vi "Comic_Crawler_Main_UI.vi"(11 "manager_daemon":refnum<class "manager_daemon.lvclass">) -> ()   [LabVIEW 2024]
uses:
  comic_crawler_class/status--cluster.ctl
  CV_downloader/status--cluster.ctl
  comic_manager/manager_daemon/manager_daemon.lvclass
  comic_crawler_class/comic_crawler.lvclass
  CV_downloader/CV_downloader.lvclass
  <vilib>/addons/_JKI Toolkits/State Machine/_JKI_lib_State_Machine.llb/Select State(s)_err__jki_lib_state_machine.vi
  003bbeb0-736b-424c-b7a2-e9a572b8fb0f.vi
  <vilib>/addons/_JKI Toolkits/State Machine/_JKI_lib_State_Machine.llb/Periodic Trigger__ogtk__JKI-SM__jki_lib_state_machine.vi
panel:
  out "added URLs":string[](array[string])
  in  "Add URL":bool
  in  "volume url":string
  out "manager status":T1
  out "size(s)":i32
  out "out of date filelist":path[](array[path])
  in  "Stop Crawler":bool
  in  "Start Crawler":bool
  out "crawler status":T2
  in  "search dirs":path[](array[path])=[path "D:/Comics/data/cv_volumes"]
  in  "Exit":bool
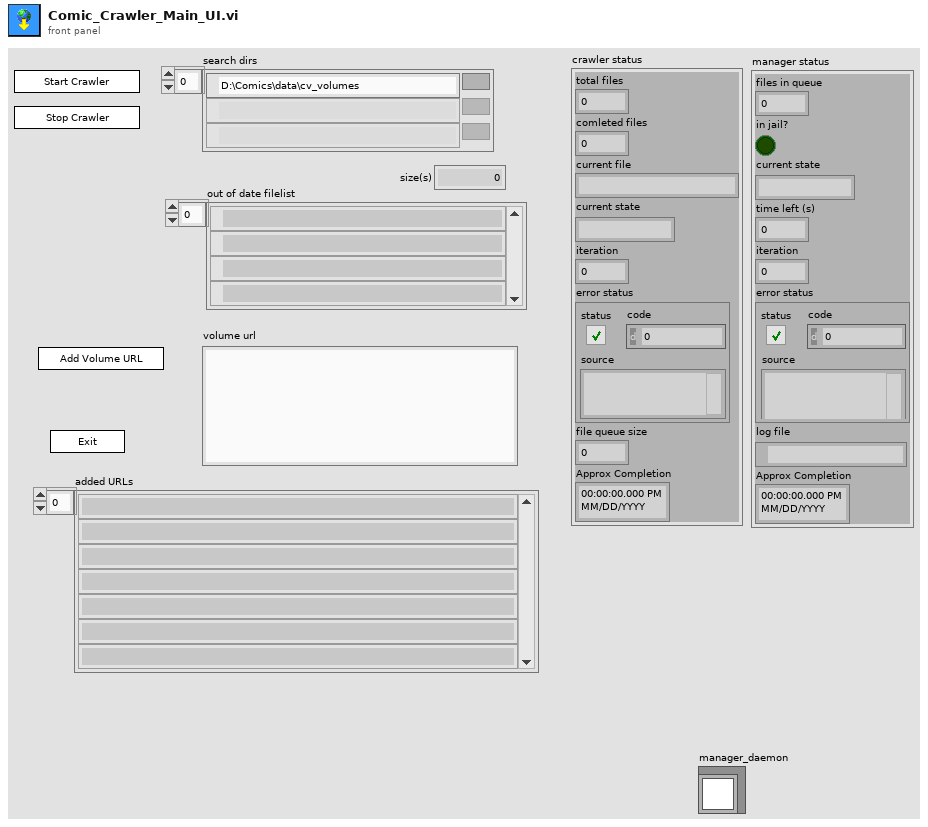
[diagram p1: front panel]
types:
  T1 = typedef "CV_downloader.lvclass/status--cluster.ctl" = cluster{"files in queue":i32, "in jail?":bool, "current state":string, "time left (s)":dbl, "iteration":i32, "error status":errorcluster, "log file":path, "Approx Completion":timestamp}
  T2 = typedef "comic_crawler.lvclass/status--cluster.ctl" = cluster{"total files":i32, "comleted files":i32, "current file":string, "current state":string, "iteration":i32, "error status":errorcluster, "file queue size":i32, "Approx Completion":timestamp}
  T3 = enum32{"Invalid", "Standard", "Closed", "Hidden", "Minimized", "Maximized"}
  T4 = enum32{"invalid app kind", "Development System", "Run Time System", "Student Edition", "Embedded LabVIEW", "Evaluation", "Custom"}
  T5 = cluster{"Core":cluster{"Current VI Reference":refnum<vi>, "Close Panel on Exit?":bool}, "TO":i32, "crawler":refnum<class "comic_crawler.lvclass">, "files for update":path[], "manager":refnum<class "CV_downloader.lvclass">, "vol_dir":path, "iss_dir":path, "manager_daemon":refnum<class "manager_daemon.lvclass">}
  T6 = cluster{"Current VI Reference":refnum<vi>, "Close Panel on Exit?":bool}
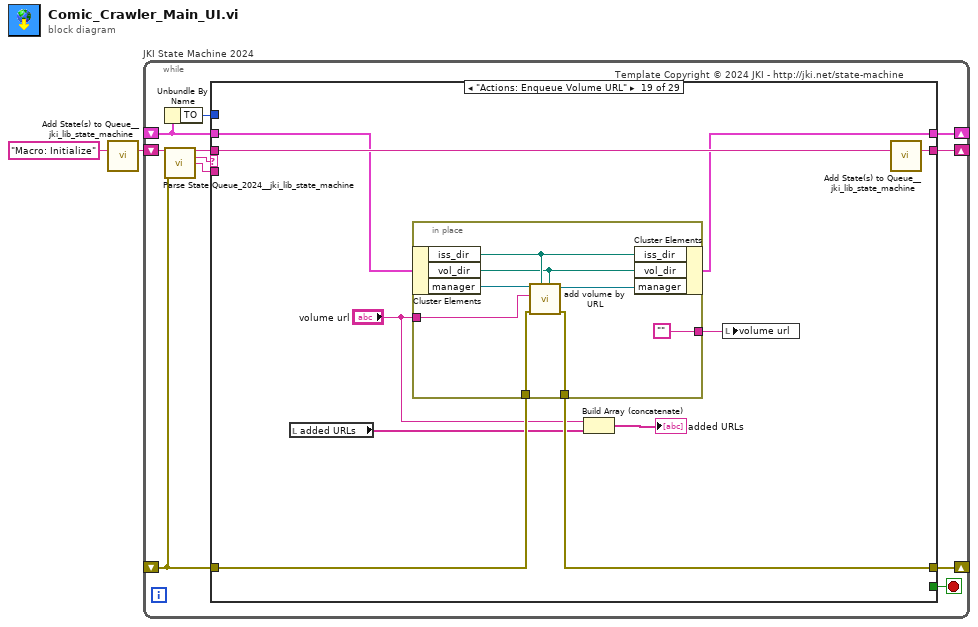
[diagram p0: block diagram]
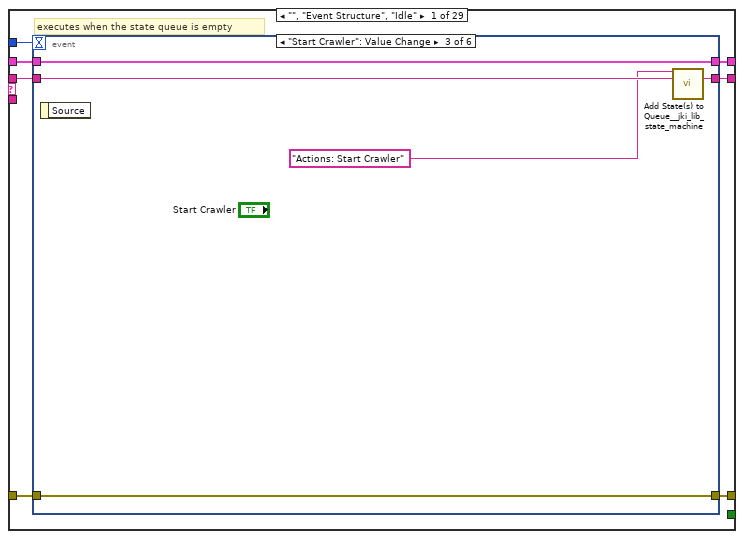
[diagram p2: hidden frame]
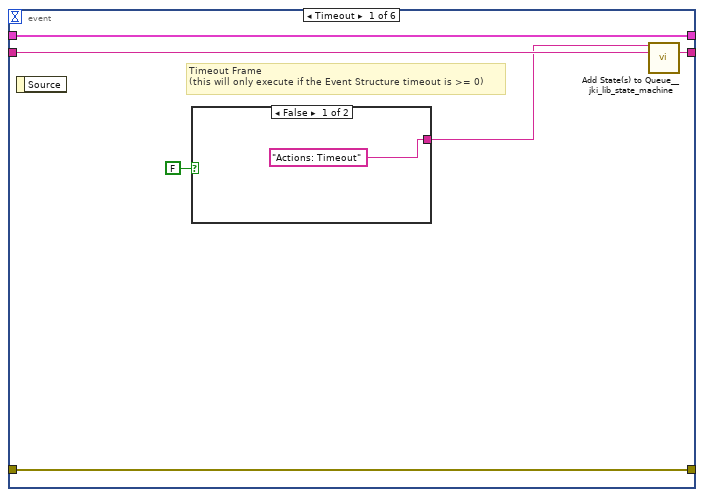
[diagram p3: hidden frame]
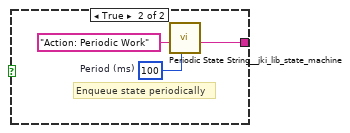
[diagram p4: hidden frame]
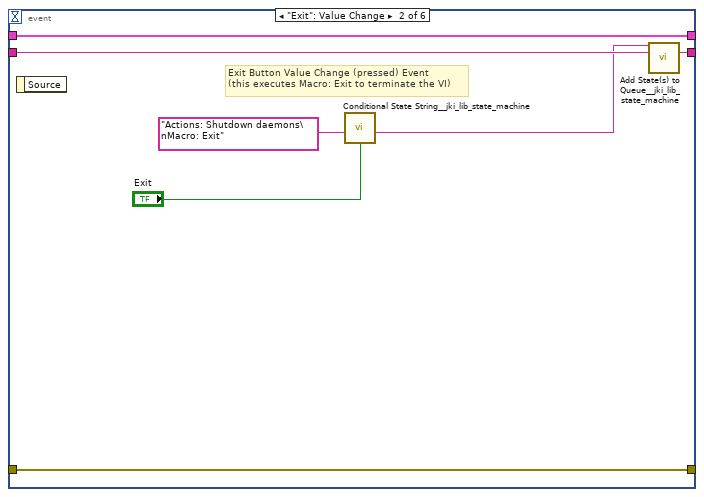
[diagram p5: hidden frame]
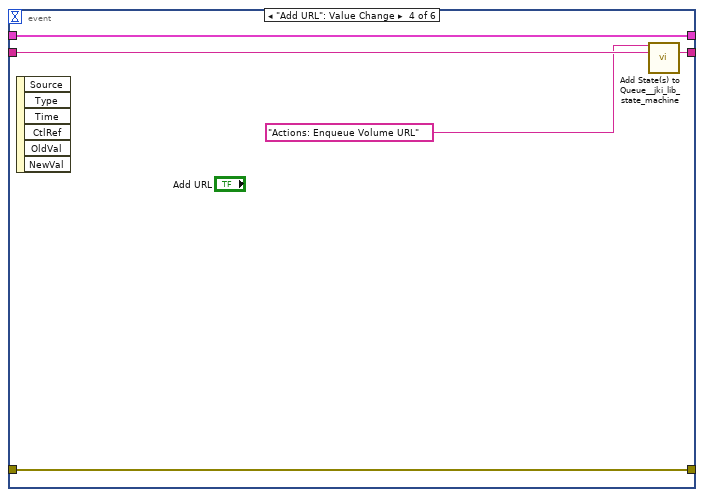
[diagram p6: hidden frame]
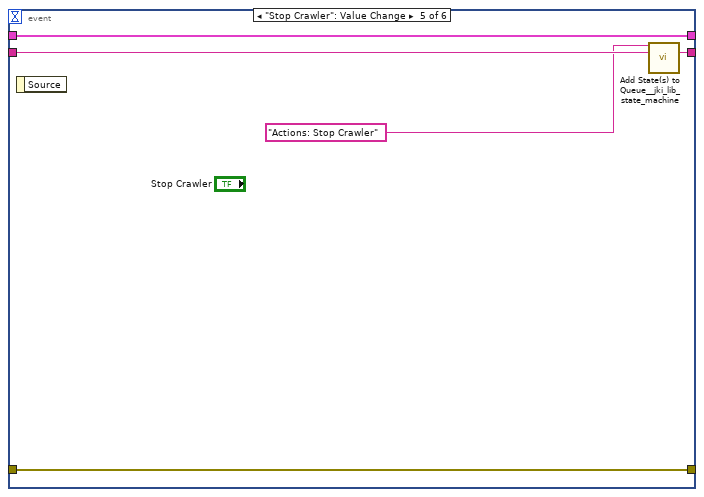
[diagram p7: hidden frame]
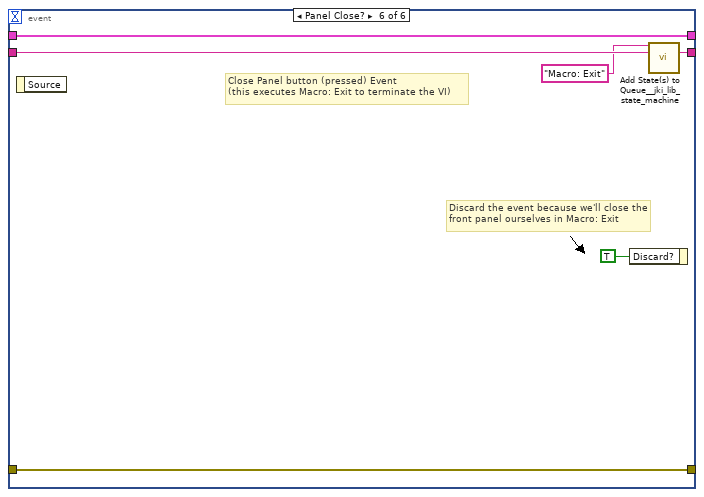
[diagram p8: hidden frame]
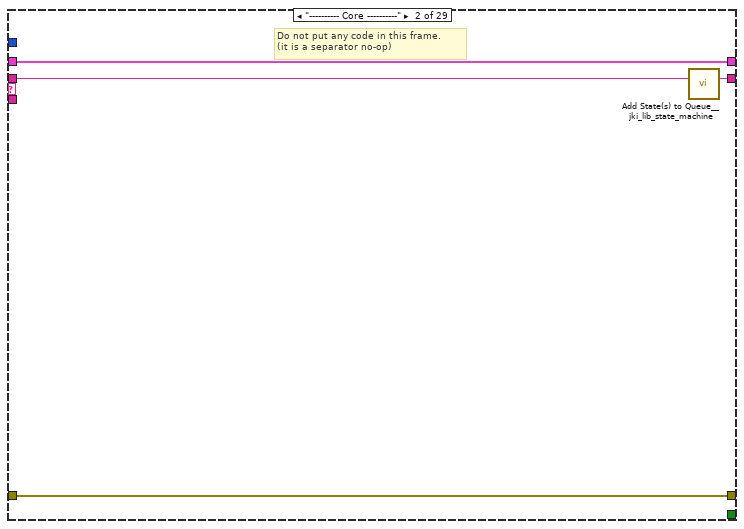
[diagram p9: hidden frame]
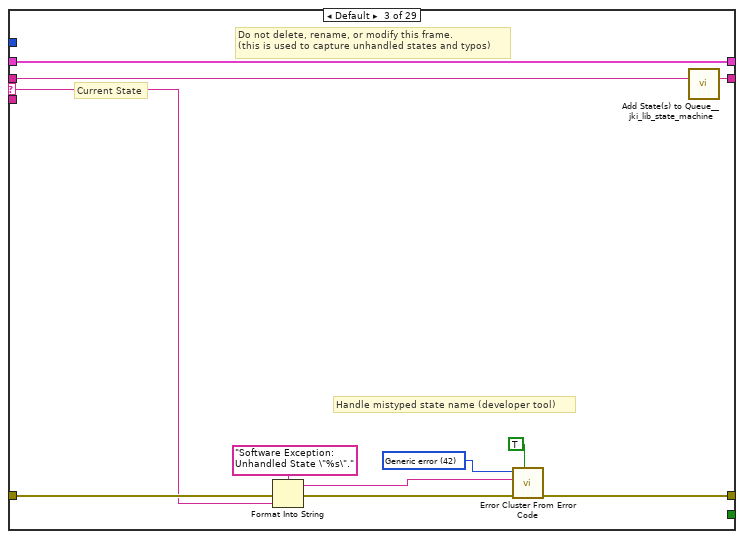
[diagram p10: hidden frame]
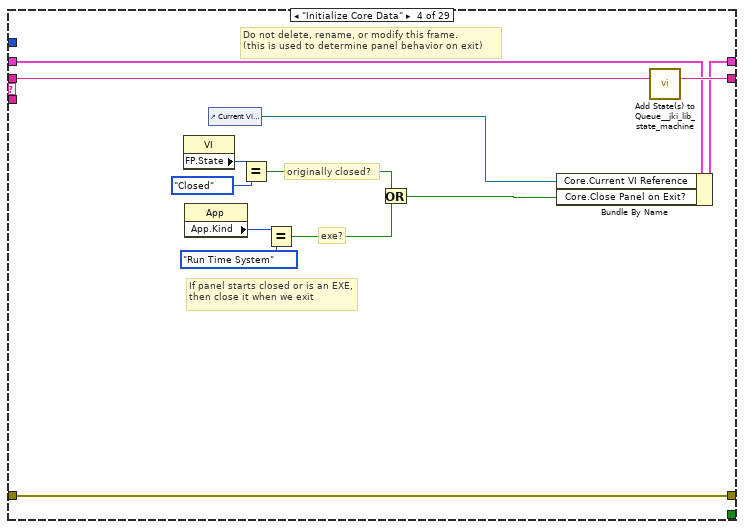
[diagram p11: hidden frame]
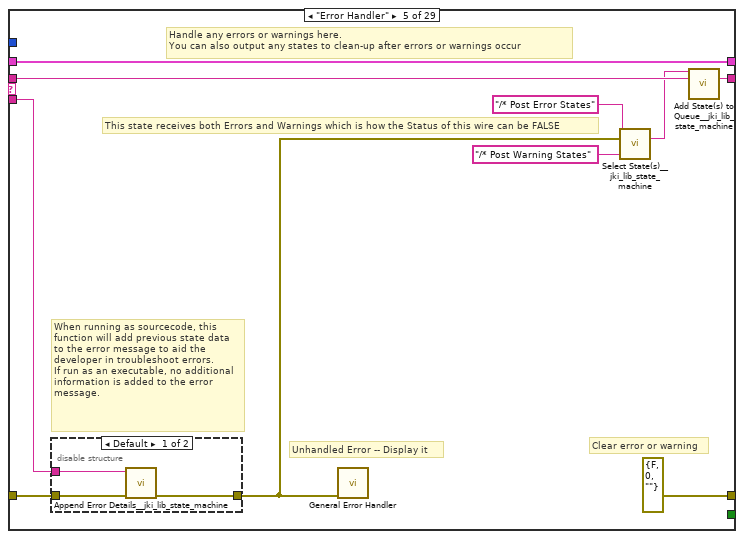
[diagram p12: hidden frame]
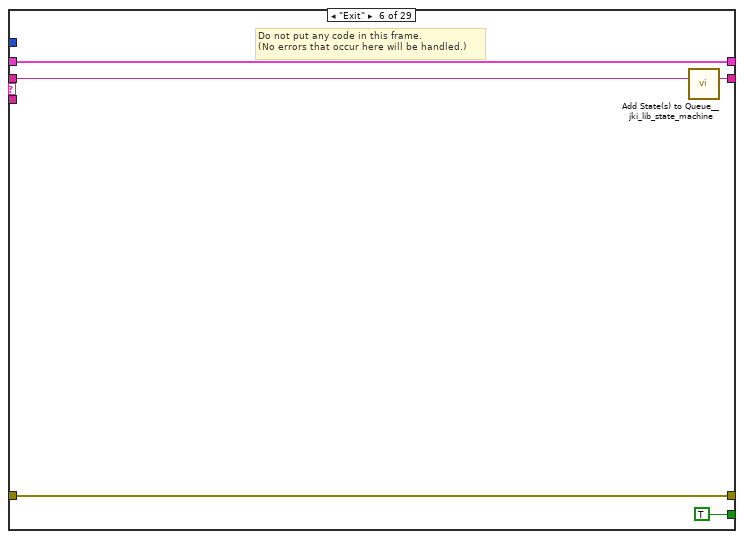
[diagram p14: hidden frame]
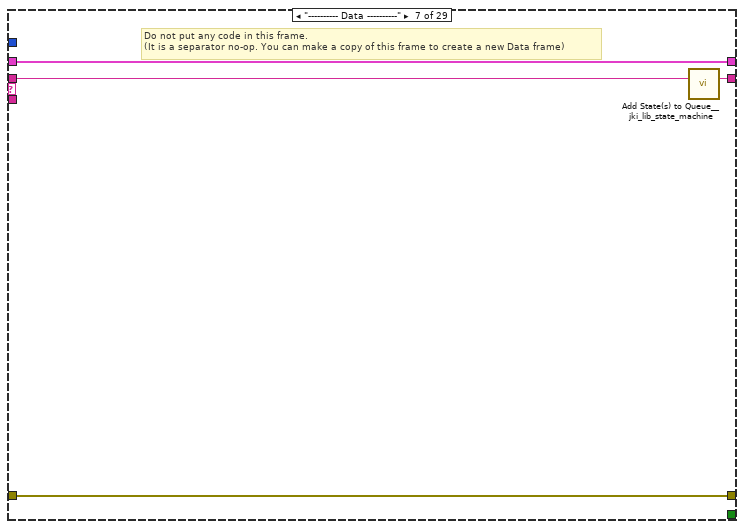
[diagram p15: hidden frame]
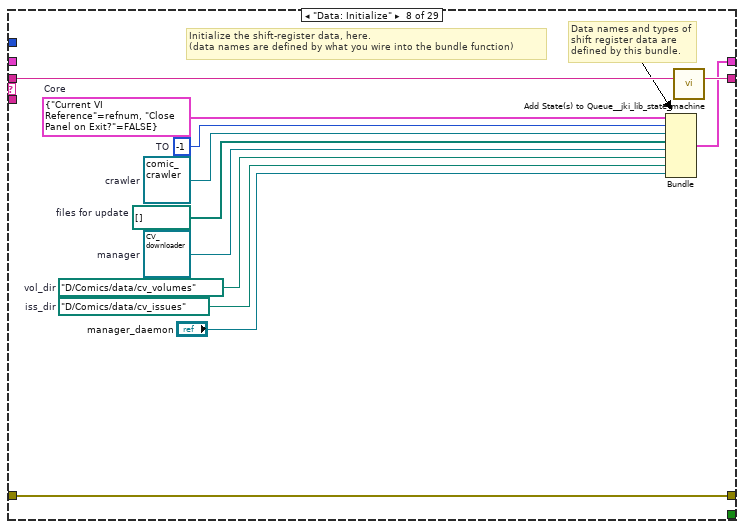
[diagram p16: hidden frame]
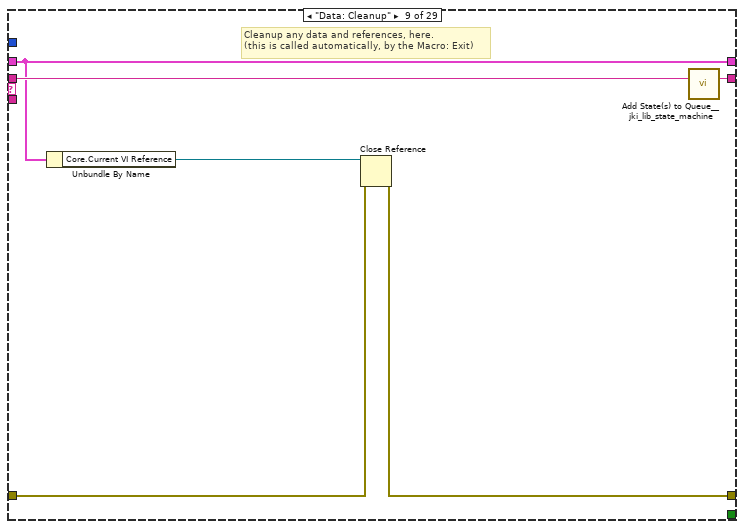
[diagram p17: hidden frame]
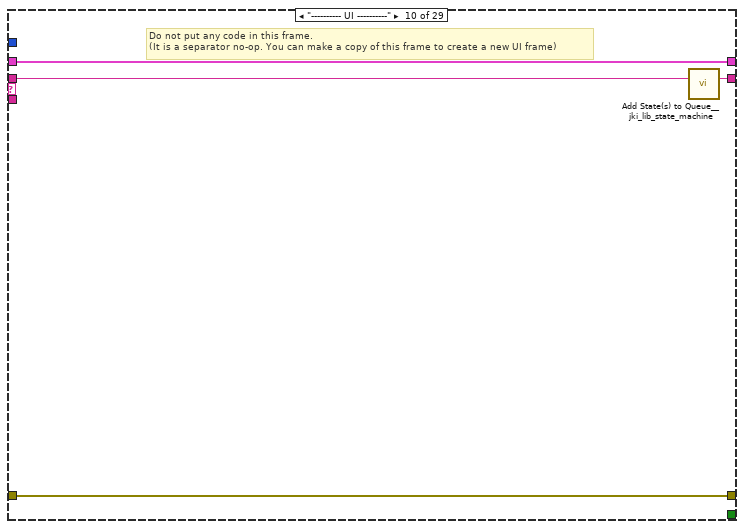
[diagram p18: hidden frame]
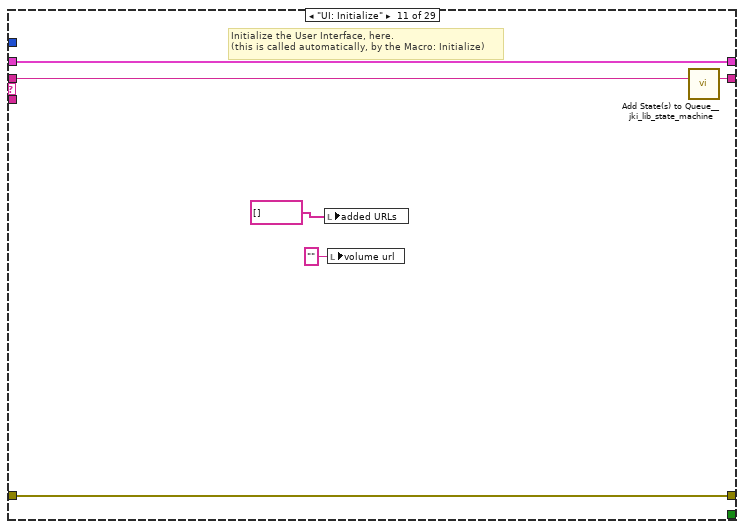
[diagram p19: hidden frame]
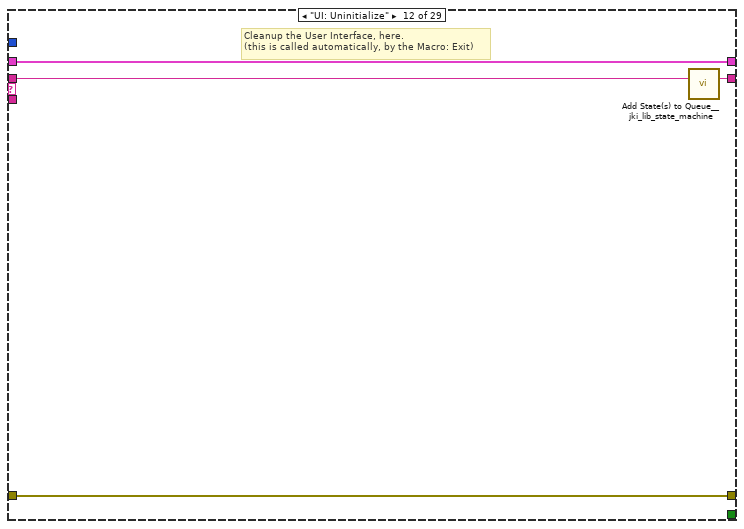
[diagram p20: hidden frame]
diagram:
  n1 = call <vilib>:"Add State(s) to Queue__jki_lib_state_machine.vi"("State(s) in (\"\")"="Macro: Initialize") -> ("States Out"=w2:string)  [unwired: 14 in]
  n2 = while "JKI State Machine 2024" {
    shift-right: [w6] -> _
    shift-left: _ -> [w4]
    shift-right: [w9] -> _
    shift-left: _ -> [w5]
    shift-right: [w8] -> _
    shift-left: w2 -> [w10]
    stop <- w7 stop-if-true
    # "Template Copyright © 2024 JKI - http://jki.net/state-machine"
    n3 = Unbundle By Name(w4) -> ("TO"=w3:i32)
    n4 = call <vilib>:"Parse State Queue_2024__jki_lib_state_machine.vi"("State Queue"=w10, "Error In (no error)"=w5) -> ("Remaining States"=w12:string, "Current State"=w13:string, "Arguments"=w11:string)  [unwired: 11 in]
    n5 = case shown="\"Actions: Enqueue Volume URL\"" w13 {
      selector: w13 -> [_ _ w63 _ _ _ _ _ _ _ _ _ _ _ _ _ _ _ _ _ _ _ _ _ _ _ _ _ _]
      tunnel: w12 -> [w20 w62 w67 w86 w96 w105 w109 w121 w127 w131 w137 w141 w147 w158 w227 w232 w241 w245 w255 w267 w276 w286 w293 w305 w318 w332 w348 w361 w373]
      tunnel: w11 -> [_ _ _ _ w91 _ _ _ _ _ _ _ w142 w152 _ _ _ _ _ _ _ _ _ _ _ _ _ _ _]
      tunnel: w4 -> [w18 w59 w65 w79 w93 w103 w106 _ w122 w128 w135 w139 w145 w154 w224 w229 w239 w242 w253 w264 w273 w280 w291 w303 w316 w330 w346 w358 w371]
      tunnel: [w17 w60 w69 w83 errorcluster {"status"=FALSE, "code"=0, "source"=""} ("error out") w102 w107 w118 w123 w129 w134 w138 w143 w155 w225 w230 w236 w243 w252 w265 w270 w282 w288 w300 w313 w325 w343 w354 w368] -> w9
      tunnel: w5 -> [w14 w60 w68 w83 w92 w102 w107 w118 w124 w129 w134 w138 w144 w156 w225 w230 w236 w243 w251 w265 w274 w283 w289 w301 w314 w328 w344 w357 w369]
      tunnel: [w19 w61 w66 w85 w95 w104 w108 w120 w126 w130 w136 w140 w146 w157 w226 w231 w240 w244 w254 w266 w275 w285 w292 w304 w317 w331 w347 w360 w372] -> w8
      tunnel: [_ _ _ _ _ TRUE _ _ _ _ _ _ _ _ _ _ _ _ _ _ _ _ _ _ _ _ _ _ _] -> w7
      tunnel: [w16 w59 w65 w84 w93 w103 w106 w119 w122 w128 w135 w139 w145 w154 w224 w229 w239 w242 w250 w264 w272 w284 w290 w302 w315 w329 w345 w358 w370] -> w6
      tunnel: w3 -> [w15 _ _ _ _ _ _ _ _ _ _ _ _ _ _ _ _ _ _ _ _ _ _ _ _ _ _ _ _]
      frame "", "Event Structure", "Idle" {
        # "executes when the state queue is empty"
        n6 = event shown="[2] \"Start Crawler\": Value Change" {
          selector: _ -> [_ _ _ _ _ _]
          dyn-events: _ -> [_ _ _ _ _ _]
          timeout: w15 -> [_ _ _ _ _ _]
          tunnel: w20 -> [w26 w37 w42 w47 w52 w58]
          tunnel: [w25 w36 w41 w46 w51 w57] -> w19
          tunnel: w18 -> [w23 w34 w39 w44 w49 w55]
          tunnel: [w24 w35 w40 w45 w50 w56] -> w17
          tunnel: w14 -> [w24 w35 w40 w45 w50 w56]
          tunnel: [w23 w34 w39 w44 w49 w55] -> w16
          event Timeout {
            # "Timeout Frame\n(this will only execute if the Event Structure timeout is >= 0)"
            n7 = event-data() -> ()  [unwired: 1 in, 1 out]
            n8 = case shown="False" FALSE {
              tunnel: ["Actions: Timeout" ("State Out") w30] -> w22
              frame False {
              }
              frame True {
                w28 = u32 100  # Period (ms)
                # "Enqueue state periodically"
                n9 = call <vilib>:"Periodic State String__jki_lib_state_machine.vi"("Period (ms)"=w28, "State"="Action: Periodic Work") -> ("State Out"=w30:string)  [unwired: 9 in]
              }
            }
            n10 = call <vilib>:"Add State(s) to Queue__jki_lib_state_machine.vi"("State(s) in Front (\"\")"=w22, "State(s) in (\"\")"=w26) -> ("States Out"=w25:string)  [unwired: 13 in]
          }
          event "Exit": Value Change {
            # "Exit Button Value Change (pressed) Event\n(this executes Macro: Exit to terminate the VI)"
            n11 = event-data() -> ()  [unwired: 1 in, 1 out]
            n12 = call <vilib>:"Conditional State String__jki_lib_state_machine.vi"("Do State(s)?"="Exit", "State"="Actions: Shutdown daemons\nMacro: Exit") -> ("State Out"=w31:string)  [unwired: 7 in]
            n13 = call <vilib>:"Add State(s) to Queue__jki_lib_state_machine.vi"("State(s) in Front (\"\")"=w31, "State(s) in (\"\")"=w37) -> ("States Out"=w36:string)  [unwired: 13 in]
          }
          event "Start Crawler": Value Change {
            n14 = event-data() -> ()  [unwired: 1 in, 1 out]
            n15 = call <vilib>:"Add State(s) to Queue__jki_lib_state_machine.vi"("State(s) in Front (\"\")"="Actions: Start Crawler", "State(s) in (\"\")"=w42) -> ("States Out"=w41:string)  [unwired: 13 in]
          }
          event "Add URL": Value Change {
            n16 = event-data() -> ()  [unwired: 1 in, 6 out]
            n17 = call <vilib>:"Add State(s) to Queue__jki_lib_state_machine.vi"("State(s) in Front (\"\")"="Actions: Enqueue Volume URL", "State(s) in (\"\")"=w47) -> ("States Out"=w46:string)  [unwired: 13 in]
          }
          event "Stop Crawler": Value Change {
            n18 = event-data() -> ()  [unwired: 1 in, 1 out]
            n19 = call <vilib>:"Add State(s) to Queue__jki_lib_state_machine.vi"("State(s) in Front (\"\")"="Actions: Stop Crawler", "State(s) in (\"\")"=w52) -> ("States Out"=w51:string)  [unwired: 13 in]
          }
          event Panel Close? {
            # "Discard the event because we'll close the front panel ourselves in Macro: Exit"
            # "Close Panel button (pressed) Event\n(this executes Macro: Exit to terminate the VI)"
            n20 = event-data() -> ()  [unwired: 1 in, 1 out]
            n21 = event-data("Discard?"=TRUE) -> ()  [unwired: 1 in, 1 out]
            n22 = call <vilib>:"Add State(s) to Queue__jki_lib_state_machine.vi"("State(s) in Front (\"\")"="Macro: Exit", "State(s) in (\"\")"=w58) -> ("States Out"=w57:string)  [unwired: 13 in]
          }
        }
      }
      frame "---------- Core ----------" {
        # "Do not put any code in this frame.\n(it is a separator no-op)"
        n23 = call <vilib>:"Add State(s) to Queue__jki_lib_state_machine.vi"("State(s) in (\"\")"=w62) -> ("States Out"=w61:string)  [unwired: 14 in]
      }
      frame Default {
        w72 = 42 items=["No error", "Argument error", "Memory is full", "Out of zone", "End of file", "File already open", "Generic file I/O error", "File not found", "File permission error", "Disk is full", "Duplicate path", "Too many files open", "System feature not enabled", "Resource file not found", "Cannot add resource", "Resource not found", "Image not found", "Image memory error", "Pen does not exist", "Config type invalid", "Config token not found", "Config parse error", "Config memory error", "Bad external code format", "Bad external code offset", "External code not present", "Null window", "Destroy window error", "Null menu", "Print aborted", "Bad print record", "Print driver error", "Windows error during printing", "Memory error during printing", "Print dialog error", "Generic print error", "Invalid device refnum", "Device not found", "Device parameter error", "Device unit error", "Cannot open device", "Device call aborted", "Generic error", "Cancelled by user", "Object ID too low", "Object ID too high", "Object not in heap", "Unknown heap", "Unknown object (invalid DefProc)", "Unknown object (DefProc not in table)", "Message out of range", "Invalid (null) method", "Unknown message", "Manager call not supported", "Bad address", "Network operation in progress", "Network operation timed out", "Connection is busy", "Network attribute not supported", "Network error", "Address in use", "System out of memory", "Connection aborted", "Connection refused", "Not connected", "Already connected", "Connection closed", "Initialization error (interapplication manager)", "Bad occurrence", "Wait on unbound occurrence handler", "Occurrence queue overflow", "Datalog type conflict", "Unused", "Unrecognized type (interapplication manager)", "Memory corrupt", "Failed to make temporary DLL", "Old CIN version", "Drag socket not found", "Failed to load drop-object", "Failed to register OLE object", "Failed to release OLE object", "Format specifier type mismatch", "Unknown format specifier", "Too few format specifiers", "Too many format specifiers", "Scan failed", "Newer CIN version", "Error converting to variant", "Runtime menu error", "Password tampered", "Variant attribute not found", "Incompatible variant data type", "Event data is not available", "Event Store is not present", "Occurrence is not found", "Event Queue is not created", "Event info is not available", "Refnum passed is NULL", "Error retrieving Class GUID", "Error retrieving CoClass GUID", "Error retrieving TypeLib GUID.", "Bad built application magic bytes.", "Specific driver is different from the specific driver associated with the Logical Name.", "There is no session opened to the class driver.", "Max Error", "MAX - Error with config objects", "MAX - Error loading configuration", "MAX - Group not supported"]
        # "Current State"
        # "Do not delete, rename, or modify this frame.\n(this is used to capture unhandled states and typos)"
        # "Handle mistyped state name (developer tool)"
        n24 = Format Into String(format string="Software Exception: Unhandled State \"%s\"." ("message"), error in=w68, w63) -> (resulting string=w71:string, error out=w70:errorcluster)  [unwired: 1 in]
        n25 = call <vilib>:"Error Cluster From Error Code.vi"("show call chain? (False)"=TRUE, "error in (no error)"=w70, "error message (\"\")"=w71, "error code (0)"=w72) -> ("error out"=w69:errorcluster)  [unwired: 5 in]
        n26 = call <vilib>:"Add State(s) to Queue__jki_lib_state_machine.vi"("State(s) in (\"\")"=w67) -> ("States Out"=w66:string)  [unwired: 14 in]
      }
      frame "Initialize Core Data" {
        # "Do not delete, rename, or modify this frame.\n(this is used to determine panel behavior on exit)"
        # "originally closed?"
        # "exe?"
        # "If panel starts closed or is an EXE, then close it when we exit"
        n27 = property class="VI"() -> ("FP.State"=w76:T3)  [unwired: 2 in, 2 out]
        n28 = property class="App"() -> ("App.Kind"=w82:T4)  [unwired: 2 in, 2 out]
        n29 = control-ref of="Current VI Reference"() -> (w77:refnum<vi>)
        n30 = Equal?(x=w76, y=T3."Closed" ("Front Panel Window:State")) -> (x = y?=w74:bool)
        n31 = Equal?(x=w82, y=T4."Run Time System" ("Application:Kind")) -> (x = y?=w80:bool)
        n32 = Or(x=w74, y=w80) -> (x .or. y?=w78:bool)
        n33 = Bundle By Name(cluster=w79, "Core.Current VI Reference"=w77, "Core.Close Panel on Exit?"=w78) -> (w84:T5)
        n34 = call <vilib>:"Add State(s) to Queue__jki_lib_state_machine.vi"("State(s) in (\"\")"=w86) -> ("States Out"=w85:string)  [unwired: 14 in]
      }
      frame "Error Handler" {
        # "When running as sourcecode, this function will add previous state data to the error message to aid the developer in troubleshoot errors.\nIf run as an executable, no additional information is added to the error message."
        # "This state receives both Errors and Warnings which is how the Status of this wire can be FALSE"
        # "Unhandled Error -- Display it"
        # "Handle any errors or warnings here.\nYou can also output any states to clean-up after errors or warnings occur"
        # "Clear error or warning"
        n35 = disable-structure shown="Default" {
          disable-tunnel: w92 -> [w99 w100]
          disable-tunnel: w91 -> [w98 _]
          disable-tunnel: [w97 w100] -> w90
          frame condition #0 (active) {
            n36 = call <vilib>:"Append Error Details__jki_lib_state_machine.vi"("error in (no error)"=w99, "Previous State and Argument(s)"=w98) -> ("error out"=w97:errorcluster)  [unwired: 9 in]
          }
          frame condition #1 {
          }
        }
        n37 = call <vilib>:"General Error Handler.vi"("error in (no error)"=w90) -> ()  [unwired: 10 in, 5 out]
        n38 = call-poly <vilib>:"Select State(s)__jki_lib_state_machine.vi"("State(s) if True (\"\")"="/* Post Error States", "Select"=w90, "State(s) if False (\"\")"="/* Post Warning States") -> ("States Out"=w88:string)  [unwired: 12 in]
        n39 = call <vilib>:"Add State(s) to Queue__jki_lib_state_machine.vi"("State(s) in Front (\"\")"=w88, "State(s) in (\"\")"=w96) -> ("States Out"=w95:string)  [unwired: 13 in]
      }
      frame "Exit" {
        # "Do not put any code in this frame.\n(No errors that occur here will be handled.)"
        n40 = call <vilib>:"Add State(s) to Queue__jki_lib_state_machine.vi"("State(s) in (\"\")"=w105) -> ("States Out"=w104:string)  [unwired: 14 in]
      }
      frame "---------- Data ----------" {
        # "Do not put any code in this frame.\n(It is a separator no-op. You can make a copy of this frame to create a new Data frame)"
        n41 = call <vilib>:"Add State(s) to Queue__jki_lib_state_machine.vi"("State(s) in (\"\")"=w109) -> ("States Out"=w108:string)  [unwired: 14 in]
      }
      frame "Data: Initialize" {
        w111 = path "D:/Comics/data/cv_issues"  # iss_dir
        w112 = path "D:/Comics/data/cv_volumes"  # vol_dir
        w113 = refnum<class "CV_downloader.lvclass"> refnum  # manager
        w114 = path[] []  # files for update
        w115 = refnum<class "comic_crawler.lvclass"> refnum  # crawler
        w116 = -1  # TO
        w117 = T6 {"Current VI Reference"=refnum, "Close Panel on Exit?"=FALSE}  # Core
        # "Data names and types of shift register data are defined by this bundle."
        # "Initialize the shift-register data, here.\n(data names are defined by what you wire into the bundle function)"
        n42 = Bundle("Core"=w117, "TO"=w116, "crawler"=w115, "files for update"=w114, "manager"=w113, "vol_dir"=w112, "iss_dir"=w111, "manager_daemon"="manager_daemon") -> (w119:T5)  [unwired: 1 in]
        n43 = call <vilib>:"Add State(s) to Queue__jki_lib_state_machine.vi"("State(s) in (\"\")"=w121) -> ("States Out"=w120:string)  [unwired: 14 in]
      }
      frame "Data: Cleanup" {
        # "Cleanup any data and references, here.\n(this is called automatically, by the Macro: Exit)"
        n44 = Unbundle By Name(w122) -> ("Core.Current VI Reference"=w125:refnum<vi>)
        n45 = Close Reference(reference=w125, error in (no error)=w124) -> (error out=w123:errorcluster)
        n46 = call <vilib>:"Add State(s) to Queue__jki_lib_state_machine.vi"("State(s) in (\"\")"=w127) -> ("States Out"=w126:string)  [unwired: 14 in]
      }
      frame "---------- UI ----------" {
        # "Do not put any code in this frame.\n(It is a separator no-op. You can make a copy of this frame to create a new UI frame)"
        n47 = call <vilib>:"Add State(s) to Queue__jki_lib_state_machine.vi"("State(s) in (\"\")"=w131) -> ("States Out"=w130:string)  [unwired: 14 in]
      }
      frame "UI: Initialize" {
        # "Initialize the User Interface, here.\n(this is called automatically, by the Macro: Initialize)"
        n48 = local write "added URLs"(string[] [] ("volume url")) -> ()
        n49 = local write "volume url"("" ("volume url")) -> ()
        n50 = call <vilib>:"Add State(s) to Queue__jki_lib_state_machine.vi"("State(s) in (\"\")"=w137) -> ("States Out"=w136:string)  [unwired: 14 in]
      }
      frame "UI: Uninitialize" {
        # "Cleanup the User Interface, here.\n(this is called automatically, by the Macro: Exit)"
        n51 = call <vilib>:"Add State(s) to Queue__jki_lib_state_machine.vi"("State(s) in (\"\")"=w141) -> ("States Out"=w140:string)  [unwired: 14 in]
      }
      frame "UI: Cursor Set" {
        # "Argument"
        # "Set and Unset Cursor Busy.\n(Usage: \"UI: Cursor Set >> Busy|Idle\")"
        n52 = case shown="\"Idle\", Default" w142 {
          tunnel: w144 -> [w149 w151]
          tunnel: [w148 w150] -> w143
          frame "Idle", Default {
            n53 = call <vilib>:"Unset Busy.vi"("error in (no error)"=w149) -> ("error out"=w148:errorcluster)  [unwired: 10 in]
          }
          frame "Busy" {
            n54 = call <vilib>:"Set Busy.vi"("error in (no error)"=w151) -> ("error out"=w150:errorcluster)  [unwired: 9 in, 1 out]
          }
        }
        n55 = call <vilib>:"Add State(s) to Queue__jki_lib_state_machine.vi"("State(s) in (\"\")"=w147) -> ("States Out"=w146:string)  [unwired: 14 in]
      }
      frame "UI: Front Panel State" {
        # "Argument"
        # "Set Front Panel Open or Closed\n(Usage: \"UI: Front Panel State >> Open|Close\")"
        n56 = Unbundle By Name(w154) -> ("Core.Current VI Reference"=w153:refnum<vi>)
        n57 = case shown="\"Minimize\", \"Minimized\"" w152 {
          tunnel: w156 -> [w164 w179 w190 w203 w216]
          tunnel: [w166 w180 w192 w205 w218] -> w155
          tunnel: w153 -> [w165 w177 w191 w204 w217]
          frame "Open", "Standard", Default {
            w159 = T3."Standard" ("State")
            n58 = property class="VI"(reference=w165, error in=w164) -> (reference out=w162:refnum<vi>, error out=w163:errorcluster, "FP.State"=w161:T3)
            n59 = Not Equal?(x=w161, y=w159) -> (x != y?=w160:bool)
            n60 = case shown="True" w160 {
              tunnel: [w170 w172] -> w166
              tunnel: w163 -> [w169 w172]
              tunnel: w162 -> [w168 _]
              tunnel: w159 -> [w167 _]
              frame True {
                n61 = invoke class="VI" method="FP.Open"(reference=w168, error in=w169, "Activate"=TRUE, "State"=w167) -> (error out=w170:errorcluster)  [unwired: 1 in, 4 out]
              }
              frame False {
              }
            }
          }
          frame "Close", "Closed" {
            n62 = property class="VI"(reference=w177, error in=w179) -> (reference out=w176:refnum<vi>, error out=w178:errorcluster, "FP.State"=w174:T3)
            n63 = Not Equal?(x=w174, y=T3."Closed" ("Front Panel Window:State")) -> (x != y?=w173:bool)
            n64 = case shown="True" w173 {
              tunnel: [w181 w184] -> w180
              tunnel: w178 -> [w181 w183]
              tunnel: w176 -> [_ w182]
              frame False {
              }
              frame True {
                n65 = invoke class="VI" method="FP.Close"(reference=w182, error in=w183) -> (error out=w184:errorcluster)  [unwired: 1 in, 2 out]
              }
            }
          }
          frame "Hidden", "Hide" {
            w185 = T3."Hidden" ("State")
            n66 = property class="VI"(reference=w191, error in=w190) -> (reference out=w188:refnum<vi>, error out=w189:errorcluster, "FP.State"=w187:T3)
            n67 = Not Equal?(x=w187, y=w185) -> (x != y?=w186:bool)
            n68 = case shown="True" w186 {
              tunnel: [w196 w197] -> w192
              tunnel: w189 -> [w195 w197]
              tunnel: w188 -> [w194 _]
              tunnel: w185 -> [w193 _]
              frame True {
                n69 = invoke class="VI" method="FP.Open"(reference=w194, error in=w195, "State"=w193) -> (error out=w196:errorcluster)  [unwired: 2 in, 4 out]
              }
              frame False {
              }
            }
          }
          frame "Minimize", "Minimized" {
            w198 = T3."Minimized" ("State")
            n70 = property class="VI"(reference=w204, error in=w203) -> (reference out=w201:refnum<vi>, error out=w202:errorcluster, "FP.State"=w200:T3)
            n71 = Not Equal?(x=w200, y=w198) -> (x != y?=w199:bool)
            n72 = case shown="True" w199 {
              tunnel: [w209 w210] -> w205
              tunnel: w202 -> [w208 w210]
              tunnel: w201 -> [w207 _]
              tunnel: w198 -> [w206 _]
              frame True {
                n73 = invoke class="VI" method="FP.Open"(reference=w207, error in=w208, "State"=w206) -> (error out=w209:errorcluster)  [unwired: 2 in, 4 out]
              }
              frame False {
              }
            }
          }
          frame "Maximize", "Maximized" {
            w211 = T3."Maximized" ("State")
            n74 = property class="VI"(reference=w217, error in=w216) -> (reference out=w214:refnum<vi>, error out=w215:errorcluster, "FP.State"=w213:T3)
            n75 = Not Equal?(x=w213, y=w211) -> (x != y?=w212:bool)
            n76 = case shown="True" w212 {
              tunnel: [w222 w223] -> w218
              tunnel: w215 -> [w221 w223]
              tunnel: w214 -> [w220 _]
              tunnel: w211 -> [w219 _]
              frame True {
                n77 = invoke class="VI" method="FP.Open"(reference=w220, error in=w221, "State"=w219) -> (error out=w222:errorcluster)  [unwired: 2 in, 4 out]
              }
              frame False {
              }
            }
          }
        }
        n78 = call <vilib>:"Add State(s) to Queue__jki_lib_state_machine.vi"("State(s) in (\"\")"=w158) -> ("States Out"=w157:string)  [unwired: 14 in]
      }
      frame "---------- Macro ----------" {
        # "Do not put any code in this frame.\n(It is a separator no-op. You can make a copy of this frame to create a new Macro frame)"
        n79 = call <vilib>:"Add State(s) to Queue__jki_lib_state_machine.vi"("State(s) in (\"\")"=w227) -> ("States Out"=w226:string)  [unwired: 14 in]
      }
      frame "Macro: Initialize" {
        w228 = "Data: Initialize\nInitialize Core Data\nUI: Initialize\nUI: Front Panel State >> Open\nActions: Create Crawler\nActions: Launch Crawler\nActions: Create Manager\nActions: Launch Manager"  # Data: Initialize Initialize Core Data UI: Initialize UI: Front Panel State >> Open Actions: Create Crawler Actions: Launch Crawler Actions: Create Manager Actions: Launch Manager
        # "Initialization Macro\n(This is called once, when the VI starts)"
        n80 = call <vilib>:"Add State(s) to Queue__jki_lib_state_machine.vi"("State(s) in Front (\"\")"=w228, "State(s) in (\"\")"=w232) -> ("States Out"=w231:string)  [unwired: 13 in]
      }
      frame "Macro: Exit" {
        # "Exit Macro\n(This is called once, when the VI exits)"
        n81 = Unbundle By Name(w239) -> ("Core.Close Panel on Exit?"=w234:bool)
        n82 = call <vilib>:"Conditional State String__jki_lib_state_machine.vi"("Do State(s)?"=w234, "State"="UI: Front Panel State >> Close") -> ("State Out"=w233:string)  [unwired: 7 in]
        n83 = call <vilib>:"Add State(s) to Queue__jki_lib_state_machine.vi"("State(s) in (\"\")"=w233, "State(s) at Back (\"\")"="UI: Uninitialize\nData: Cleanup\nExit") -> ("States Out"=w237:string)  [unwired: 13 in]
        n84 = call <vilib>:"Add State(s) to Queue__jki_lib_state_machine.vi"("State(s) in Front (\"\")"=w237, "State(s) in (\"\")"=w241) -> ("States Out"=w240:string)  [unwired: 13 in]
      }
      frame "---------- Actions ----------" {
        # "Template Separator\n(You can make a copy of, or modify, this frame)"
        n85 = call <vilib>:"Add State(s) to Queue__jki_lib_state_machine.vi"("State(s) in (\"\")"=w245) -> ("States Out"=w244:string)  [unwired: 14 in]
      }
      frame "Actions: Enqueue Volume URL" {
        n86 = local read "added URLs"() -> (w249:string[])
        n87 = in-place {
          in-place-border: w251 -> [w261]
          in-place-border: [w260] -> w252
          in-place-border: "volume url" -> [w257]
          in-place-border: [""] -> w247
          n88 = in-place-cluster #1(w253) -> ("iss_dir"=w259:path, "vol_dir"=w258:path, "manager"=w263:refnum<class "CV_downloader.lvclass">)
          n89 = call "add volume by URL.vi"("volume parent dir"=w258, "issue parent dir"=w259, "error in (no error)"=w261, "URL"=w257, "ComicVine_manager in"=w263) -> ("error out"=w260:errorcluster, "ComicVine_manager out"=w262:refnum<class "CV_downloader.lvclass">)  [unwired: 5 in]
          n90 = in-place-cluster #1("iss_dir"=w259, "vol_dir"=w258, "manager"=w262) -> (w250:T5)
        }
        n91 = Build Array (concatenate)("volume url", w249) -> (→"added URLs":string[])
        n92 = local write "volume url"(w247) -> ()
        n93 = call <vilib>:"Add State(s) to Queue__jki_lib_state_machine.vi"("State(s) in (\"\")"=w255) -> ("States Out"=w254:string)  [unwired: 14 in]
      }
      frame "Actions: Periodic Action" {
        n94 = call <vilib>:"Add State(s) to Queue__jki_lib_state_machine.vi"("State(s) in (\"\")"=w267) -> ("States Out"=w266:string)  [unwired: 14 in]
      }
      frame "Actions: Create Crawler" {
        n95 = call "create.vi"("error in"=w274, "delay (s)"=2.0) -> ("error out"=w270:errorcluster, "comic_crawler.lvclass"=w271:refnum<class "comic_crawler.lvclass">)  [unwired: 8 in]
        n96 = Bundle By Name(cluster=w273, "TO"=-1, "crawler"=w271) -> (w272:T5)
        n97 = call <vilib>:"Add State(s) to Queue__jki_lib_state_machine.vi"("State(s) in (\"\")"=w276) -> ("States Out"=w275:string)  [unwired: 14 in]
      }
      frame "Actions: Create Manager" {
        n98 = Unbundle By Name(w280) -> ("vol_dir"=w279:path, "iss_dir"=w278:path, "manager_daemon"=w277:refnum<class "manager_daemon.lvclass">)
        n99 = call "create.vi"("error in (no error)"=w283, "manager_daemon"=w277, "issue directory"=w278, "volume directory"=w279) -> ("error out"=w282:errorcluster, "ComicVine_manager out"=w281:refnum<class "CV_downloader.lvclass">)  [unwired: 6 in]
        n100 = Bundle By Name(cluster=w280, "manager"=w281) -> (w284:T5)
        n101 = call <vilib>:"Add State(s) to Queue__jki_lib_state_machine.vi"("State(s) in (\"\")"=w286) -> ("States Out"=w285:string)  [unwired: 14 in]
      }
      frame "Actions: Launch Crawler" {
        n102 = in-place {
          in-place-border: w289 -> [w296]
          in-place-border: [w295] -> w288
          in-place-border: 100 ("Tester Timeout") -> [w294]
          n103 = in-place-cluster #2(w291) -> ("crawler"=w298:refnum<class "comic_crawler.lvclass">)  [unwired: 1 out]
          n104 = call "Launch.vi"("error in (no error)"=w296, "comic_crawler in"=w298) -> ("error out"=w295:errorcluster, "comic_crawler out"=w297:refnum<class "comic_crawler.lvclass">)  [unwired: 8 in]
          n105 = in-place-cluster #2("crawler"=w297, "TO"=w294) -> (w290:T5)
        }
        n106 = call <vilib>:"Add State(s) to Queue__jki_lib_state_machine.vi"("State(s) in (\"\")"=w293) -> ("States Out"=w292:string)  [unwired: 14 in]
      }
      frame "Actions: Launch Manager" {
        n107 = in-place {
          in-place-border: w301 -> [w307]
          in-place-border: [w306] -> w300
          in-place-border: 100 ("Tester Timeout") -> [w310]
          n108 = in-place-cluster #3(w303) -> ("manager"=w309:refnum<class "CV_downloader.lvclass">)  [unwired: 1 out]
          n109 = call "Launch.vi"("error in (no error)"=w307, "ComicVine_manager in"=w309) -> ("error out"=w306:errorcluster, "ComicVine_manager out"=w308:refnum<class "CV_downloader.lvclass">)  [unwired: 8 in]
          n110 = in-place-cluster #3("manager"=w308, "TO"=w310) -> (w302:T5)
        }
        n111 = call <vilib>:"Add State(s) to Queue__jki_lib_state_machine.vi"("State(s) in (\"\")"=w305) -> ("States Out"=w304:string)  [unwired: 14 in]
      }
      frame "Actions: Start Crawler" {
        n112 = in-place {
          in-place-border: w314 -> [w322]
          in-place-border: [w321] -> w313
          in-place-border: "search dirs" -> [w320]
          in-place-border: [w319] -> w311
          w319 = path[] [] ("files for update")
          n113 = in-place-cluster #4(w316) -> ("crawler"=w324:refnum<class "comic_crawler.lvclass">)  [unwired: 1 out]
          n114 = call "Start.vi"("error in (no error)"=w322, "search dirs"=w320, "comic_crawler in"=w324) -> ("error out"=w321:errorcluster, "comic_crawler out"=w323:refnum<class "comic_crawler.lvclass">)  [unwired: 7 in]
          n115 = in-place-cluster #4("files for update"=w319, "crawler"=w323) -> (w315:T5)
        }
        "out of date filelist" <- w311
        n116 = call <vilib>:"Add State(s) to Queue__jki_lib_state_machine.vi"("State(s) in (\"\")"=w318) -> ("States Out"=w317:string)  [unwired: 14 in]
      }
      frame "Actions: Get Filelist" {
        n117 = in-place {
          in-place-border: w328 -> [w340]
          in-place-border: [w338] -> w327
          in-place-border: [w333] -> w325
          n118 = in-place-cluster #5(w330) -> ("manager"=w335:refnum<class "CV_downloader.lvclass">, "files for update"=w339:path[], "crawler"=w342:refnum<class "comic_crawler.lvclass">)
          n119 = call "Filelist.get.vi"("error in (no error)"=w340, "comic_crawler in"=w342) -> ("error out"=w336:errorcluster, "out of date filelist"=w337:path[], "comic_crawler out"=w341:refnum<class "comic_crawler.lvclass">)  [unwired: 7 in]
          n120 = call "add filepath array.vi"("error in (no error)"=w336, "filepath array"=w337, "ComicVine_manager in"=w335) -> ("error out"=w333:errorcluster, "ComicVine_manager out"=w334:refnum<class "CV_downloader.lvclass">)  [unwired: 7 in]
          n121 = Build Array (concatenate)(w339, w337) -> (w338:path[])
          n122 = in-place-cluster #5("manager"=w334, "files for update"=w338, "crawler"=w341) -> (w329:T5)
        }
        n123 = local write "out of date filelist"(w327) -> ()
        n124 = Array Size(array=w327) -> (size(s)=→"size(s)":i32)
        n125 = call <vilib>:"Add State(s) to Queue__jki_lib_state_machine.vi"("State(s) in (\"\")"=w332) -> ("States Out"=w331:string)  [unwired: 14 in]
      }
      frame "Actions: Stop Crawler" {
        n126 = in-place {
          in-place-border: w344 -> [w350]
          in-place-border: [w349] -> w343
          n127 = in-place-cluster #6(w346) -> ("crawler"=w352:refnum<class "comic_crawler.lvclass">)
          n128 = call "Stop.vi"("error in (no error)"=w350, "comic_crawler in"=w352) -> ("error out"=w349:errorcluster, "comic_crawler out"=w351:refnum<class "comic_crawler.lvclass">)  [unwired: 8 in]
          n129 = in-place-cluster #6("crawler"=w351) -> (w345:T5)
        }
        n130 = call <vilib>:"Add State(s) to Queue__jki_lib_state_machine.vi"("State(s) in (\"\")"=w348) -> ("States Out"=w347:string)  [unwired: 14 in]
      }
      frame "Actions: Shutdown daemons" {
        n131 = Unbundle By Name(w358) -> ("manager"=w353:refnum<class "CV_downloader.lvclass">, "crawler"=w359:refnum<class "comic_crawler.lvclass">)
        n132 = call "destroy.vi"("comic_crawler in"=w359) -> ("error out"=w355:errorcluster)  [unwired: 10 in]
        n133 = call "destroy.vi"("ComicVine_manager in"=w353) -> ("error out"=w356:errorcluster)  [unwired: 10 in]
        n134 = Merge Errors(w357, w356, w355) -> (w354:errorcluster)
        n135 = call <vilib>:"Add State(s) to Queue__jki_lib_state_machine.vi"("State(s) in (\"\")"=w361) -> ("States Out"=w360:string)  [unwired: 14 in]
      }
      frame "Actions: Timeout" {
        n136 = in-place {
          in-place-border: [w381] -> w366
          in-place-border: w369 -> [w379]
          in-place-border: [w375] -> w368
          in-place-border: [w374] -> w362
          n137 = in-place-cluster #7(w371) -> ("manager"=w378:refnum<class "CV_downloader.lvclass">, "crawler"=w382:refnum<class "comic_crawler.lvclass">)
          n138 = call "Status.get.vi"("error in (no error)"=w379, "comic_crawler in"=w382) -> ("error out"=w376:errorcluster, "current status"=w381:T2, "comic_crawler out"=w380:refnum<class "comic_crawler.lvclass">)  [unwired: 7 in]
          n139 = call "Status.get.vi"("error in (no error)"=w376, "ComicVine_manager in"=w378) -> ("error out"=w375:errorcluster, "current status"=w374:T1, "ComicVine_manager out"=w377:refnum<class "CV_downloader.lvclass">)  [unwired: 7 in]
          n140 = in-place-cluster #7("manager"=w377, "crawler"=w380) -> (w370:T5)
        }
        "crawler status" <- w366
        "manager status" <- w362
        n141 = Unbundle By Name(w366) -> ("file queue size"=w367:i32)
        n142 = call "Is Value Changed.vim"("value"=w367) -> ("changed or first call?"=w365:bool)
        n143 = call <vilib>:"Conditional State String__jki_lib_state_machine.vi"("Do State(s)?"=w365, "State"="Actions: Get Filelist") -> ("State Out"=w364:string)  [unwired: 7 in]
        n144 = call <vilib>:"Add State(s) to Queue__jki_lib_state_machine.vi"("State(s) in Front (\"\")"=w364, "State(s) in (\"\")"=w373) -> ("States Out"=w372:string)  [unwired: 13 in]
      }
    }
  }
